vi "ActionVIOnDownload_Good.vi"(5 "System Definition Dir":path, 6 "IP address":string, 7 "Details Ref":refnum<vi>, 8 "error in (no error)":errorcluster, 10 "WebDAV session in":T1, 11 "Device Item Ref in":T2 format="%.0x") -> (0 "error out":errorcluster, 2 "WebDAV session out":T1, 3 "Device Item Ref out":T2 format="%.0x")   [LabVIEW 2027]
uses:
  <vilib>/NI VeriStand/Custom Device API/Custom Device Item Ref.ctl
  <vilib>/WebDAVClient/Advanced/SessionHandle.ctl
  <vilib>/NI VeriStand/Custom Device API/Custom Device API.lvlib
  <vilib>/WebDAVClient/NI_WebDAV.lvlib
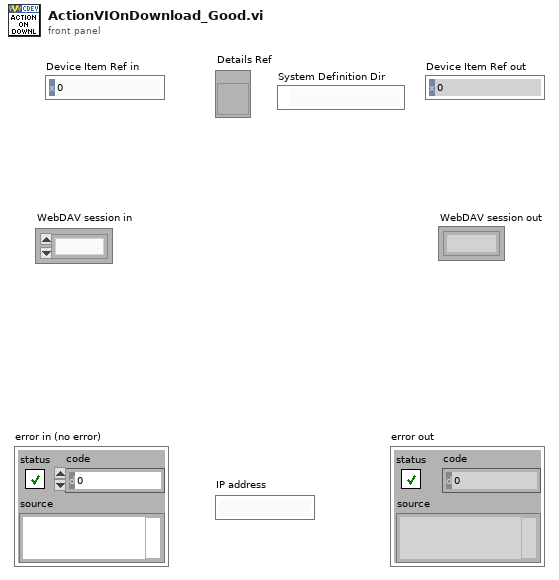
[diagram p1: front panel]
types:
  T1 = typedef "NI_WebDAV.lvlib/SessionHandle.ctl" = refnum<k1>
  T2 = typedef "Custom Device API.lvlib/Custom Device Item Ref.ctl" = u64
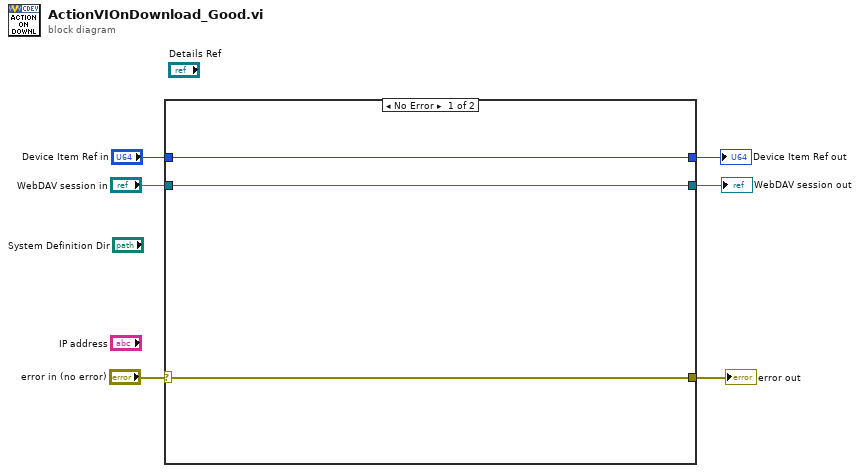
[diagram p0: block diagram]
diagram:
  n1 = case shown="No Error" "error in (no error)" {
    selector: "error in (no error)" -> [w9 w12]
    tunnel: [w9 w12] -> w5
    tunnel: "WebDAV session in" -> [w8 w11]
    tunnel: [w8 w11] -> w1
    tunnel: "Device Item Ref in" -> [w7 w10]
    tunnel: [w7 w10] -> w3
    frame No Error {
    }
    frame Error {
    }
  }
  "error out" <- w5
  "Device Item Ref out" <- w3
  "WebDAV session out" <- w1
